vi "Delta_Hz.vi"(1 "Counts":u32[](array[numeric])=[0, 0, 0, 0, 0, 0, 0, 0]) -> (0 "Delta":i32[](array[numeric]))   [LabVIEW 2014]
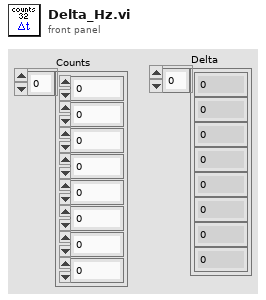
[diagram p1: front panel]
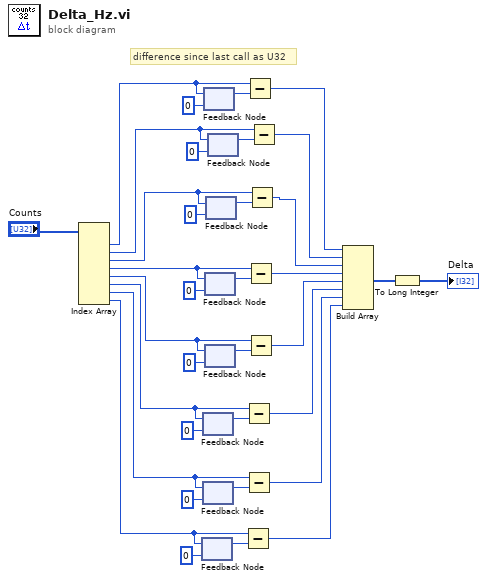
[diagram p0: block diagram]
diagram:
  # "difference since last call as U32"
  n1 = Index Array(array="Counts") -> (element #1=w26:u32, element #2=w25:u32, element #3=w24:u32, element #4=w23:u32, element #5=w22:u32, element #6=w21:u32, element #7=w20:u32, element #8=w19:u32)  [unwired: 8 in]
  n2 = feedback #1(u32 0 ("element")) -> (w28:u32)
  n3 = feedback-in #1(w19) -> ()
  n4 = feedback #2(u32 0 ("element")) -> (w30:u32)
  n5 = feedback-in #2(w21) -> ()
  n6 = feedback #3(u32 0 ("element")) -> (w29:u32)
  n7 = feedback-in #3(w20) -> ()
  n8 = feedback-in #4(w26) -> ()
  n9 = feedback #4(u32 0 ("element")) -> (w35:u32)
  n10 = feedback #5(u32 0 ("element")) -> (w32:u32)
  n11 = feedback-in #5(w23) -> ()
  n12 = feedback #6(u32 0 ("element")) -> (w31:u32)
  n13 = feedback-in #6(w22) -> ()
  n14 = feedback #7(u32 0 ("element")) -> (w33:u32)
  n15 = feedback-in #7(w24) -> ()
  n16 = feedback #8(u32 0 ("element")) -> (w34:u32)
  n17 = feedback-in #8(w25) -> ()
  n18 = Subtract(x=w19, y=w28) -> (x-y=w3:u32)
  n19 = Subtract(x=w21, y=w30) -> (x-y=w5:u32)
  n20 = Subtract(x=w20, y=w29) -> (x-y=w4:u32)
  n21 = Subtract(x=w26, y=w35) -> (x-y=w10:u32)
  n22 = Subtract(x=w23, y=w32) -> (x-y=w7:u32)
  n23 = Subtract(x=w22, y=w31) -> (x-y=w6:u32)
  n24 = Subtract(x=w24, y=w33) -> (x-y=w8:u32)
  n25 = Subtract(x=w25, y=w34) -> (x-y=w9:u32)
  n26 = Build Array(w10, w9, w8, w7, w6, w5, w4, w3) -> (w2:u32[])
  n27 = To Long Integer(number=w2) -> (32bit integer=→"Delta":i32[])
